vi "SetConfig.vi"(8 "error in (no error)":errorcluster, 10 "Variant":variant, 11 "PmuTestFunctions in":refnum<class "PmuTestFunctions.lvclass">) -> (0 "error out":errorcluster, 3 "PmuTestFunctions out":refnum<class "PmuTestFunctions.lvclass">)   [LabVIEW 2018, in "Functions.lvlib" / "PmuTestFunctions.lvclass"]
uses:
  PmuTestFunctions.lvclass
  PmuTestConfig.ctl
  ArbitraryFunction/TypeDefs/ArbCfg.ctl
  ArbitraryFunction/TypeDefs/Arbitrary.ctl
  PmuTestFunctions.lvclass/PmuTestFunctions.ctl
  Accessors/Write T0.vi
  Accessors/Write SettlingTime.vi
  ArbitraryFunction/ArbitraryFunction.lvclass
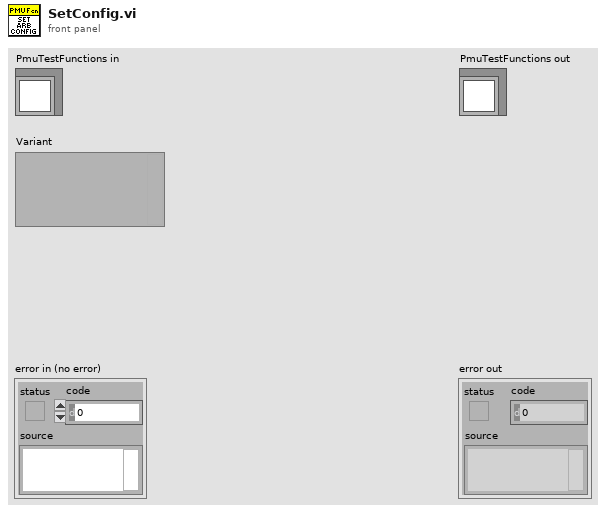
[diagram p1: front panel]
types:
  T1 = typedef "Functions.lvlib/PmuTestFunctions.lvclass/PmuTestConfig.ctl" = cluster{"T0":dbl, "SettlingTime":dbl, "ArbCfg":T2}
  T2 = typedef "Functions.lvlib/ArbitraryFunction.lvclass/ArbCfg.ctl" = cluster{"SampleRate":dbl, "Count":u16, "Arbs":T3[]}
  T3 = typedef "Functions.lvlib/ArbitraryFunction.lvclass/Arbitrary.ctl" = cluster{"Handle":string, "Size":i32, "Gain":dbl, "Offset":dbl, "Waveform":waveform(dbl)}
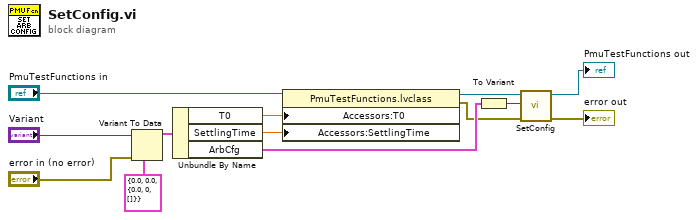
[diagram p0: block diagram]
diagram:
  n1 = Variant To Data(error in="error in (no error)", type=T1 {"T0"=0.0, "SettlingTime"=0.0, "ArbCfg"={"SampleRate"=0.0, "Count"=0, "Arbs"=[]}} ("PmuTestConfig"), Variant="Variant") -> (data=w7:T1)  [unwired: 1 out]
  n2 = Unbundle By Name(w7) -> ("T0"=w3:dbl, "SettlingTime"=w2:dbl, "ArbCfg"=w5:T2)
  n3 = property class="PmuTestFunctions.lvclass"(reference="PmuTestFunctions in", "Accessors:T0"=w3, "Accessors:SettlingTime"=w2) -> (reference out=w4:refnum<class "PmuTestFunctions.lvclass">, error out=w1:errorcluster)  [unwired: 1 in]
  n4 = To Variant(anything=w5) -> (Variant=w6:variant)
  n5 = call-parent "SetConfig.vi"("error in (no error)"=w1, "Variant"=w6, "ArbitraryFunction in"=w4) -> ("error out"=→"error out":errorcluster, "ArbitraryFunction out"=→"PmuTestFunctions out":refnum<class "PmuTestFunctions.lvclass">)  [unwired: 7 in]
